vi "RDV-preLaunchConfig.vi"(8 "error in (no error)":errorcluster, 10 "preLaunch Config":T1, 11 "RDV-Reflection_Data_viewer in":refnum<class "RDV-Reflection_Data_viewer.lvclass">) -> (0 "error out":errorcluster, 3 "RDV-Reflection_Data_viewer out":refnum<class "RDV-Reflection_Data_viewer.lvclass">)   [LabVIEW 2020, in "RDV-Reflection_Data_viewer.lvclass"]
uses:
  RDV-Reflection_Data_viewer.lvclass
  RDV-PRELAUNCH_DATA.ctl
  RDV-XY_GRAPH_REFS.ctl
  RDV-Reflection_Data_viewer.lvclass/RDV-Reflection_Data_viewer.ctl
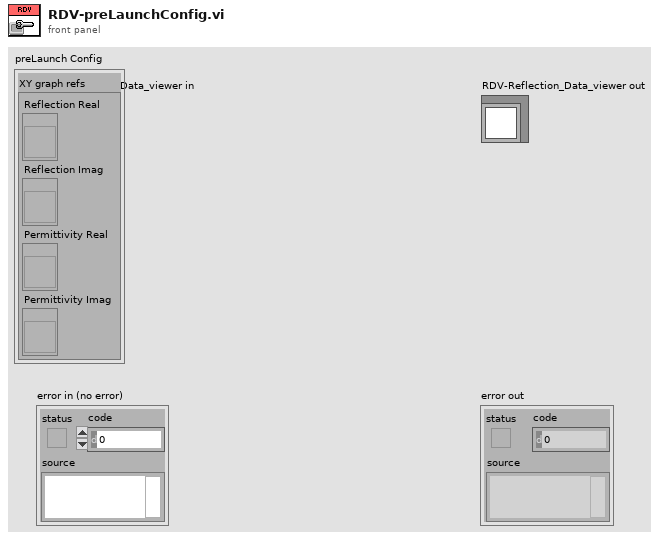
[diagram p1: front panel]
types:
  T1 = typedef "RDV-Reflection_Data_viewer.lvclass/RDV-PRELAUNCH_DATA.ctl" = cluster{"XY graph refs":T2}
  T2 = typedef "RDV-Reflection_Data_viewer.lvclass/RDV-XY_GRAPH_REFS.ctl" = cluster{"Reflection Real":refnum<vi>, "Reflection Imag":refnum<vi>, "Permittivity Real":refnum<vi>, "Permittivity Imag":refnum<vi>}
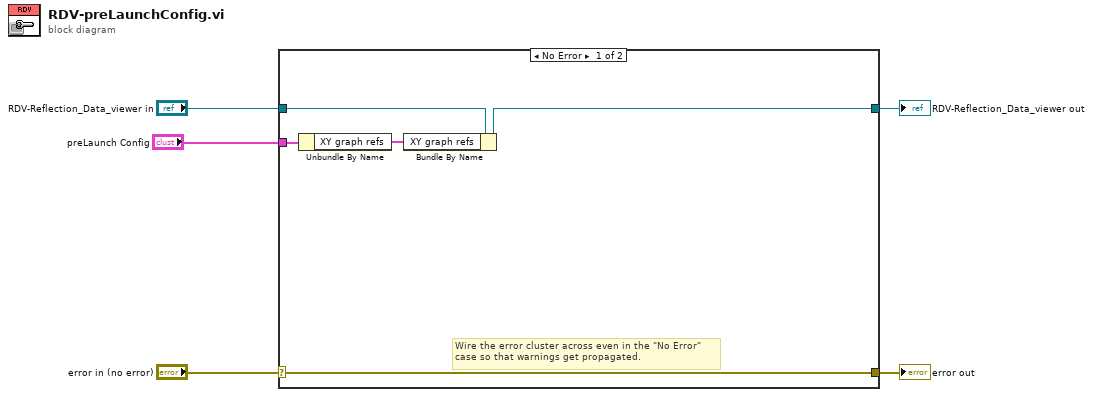
[diagram p0: block diagram]
diagram:
  n1 = case shown="No Error" "error in (no error)" {
    selector: "error in (no error)" -> [w9 w12]
    tunnel: [w9 w12] -> w4
    tunnel: [w7 w11] -> w2
    tunnel: "RDV-Reflection_Data_viewer in" -> [w10 w11]
    tunnel: "preLaunch Config" -> [w8 _]
    frame No Error {
      # "Wire the error cluster across even in the \"No Error\"\ncase so that warnings get propagated."
      n2 = Unbundle By Name(w8) -> ("XY graph refs"=w6:T2)
      n3 = Bundle By Name(cluster=w10, "XY graph refs"=w6) -> (w7:refnum<class "RDV-Reflection_Data_viewer.lvclass">)
    }
    frame Error {
    }
  }
  "error out" <- w4
  "RDV-Reflection_Data_viewer out" <- w2
